vi "Value Set Callback.vi"(8 "error in (no error)":errorcluster, 9 "Scope":variant, 11 "Value":variant) -> (0 "error out":errorcluster)   [LabVIEW 2017, in "Promise Future.lvlib" / "Future.lvclass"]
uses:
  Future.lvclass
  Future.lvclass/Future.ctl
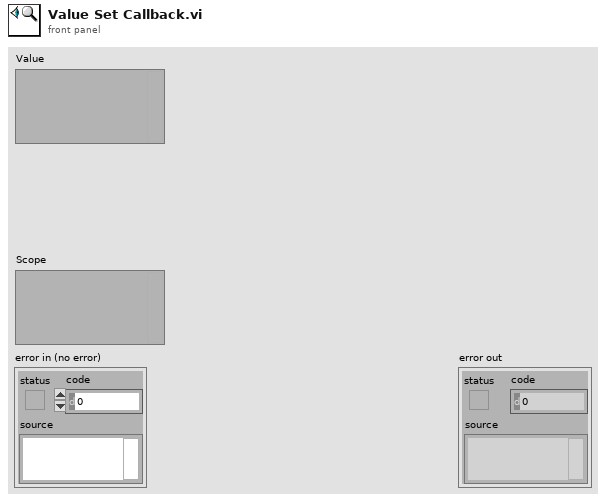
[diagram p1: front panel]
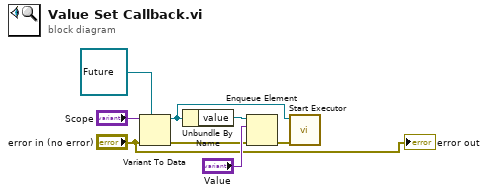
[diagram p0: block diagram]
diagram:
  n1 = Variant To Data(error in="error in (no error)", type=refnum<class "Future.lvclass"> refnum ("Promise Future.lvlib:Future.lvclass"), Variant="Scope") -> (data=w5:refnum<class "Future.lvclass">, error out=w3:errorcluster)
  n2 = Unbundle By Name(w5) -> ("value"=w6:refnum<queue>)
  n3 = Enqueue Element(queue=w6, element="Value", error in (no error)=w3) -> (error out=w2:errorcluster)  [unwired: 1 in, 2 out]
  n4 = call "Start Executor.vi"("error in (no error)"=w2, "Future in"=w5) -> ()  [unwired: 8 in, 2 out]
  "error out" <- "error in (no error)"
